vi "INI Create Semaphore.vi"(4 "error in":errorcluster) -> (0 "error out":errorcluster, 3 "semaphore":T1)   [LabVIEW 2013]
doc: "Produces the .ini semaphore that restricts reading/writing to the .ini file."
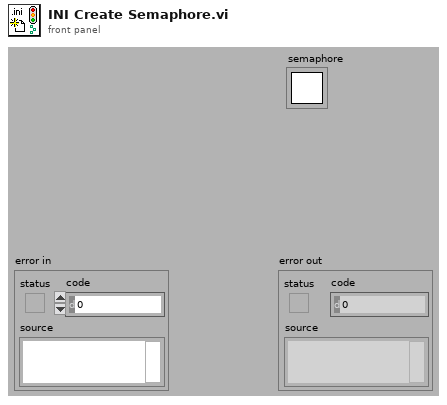
[diagram p1: front panel]
types:
  T1 = typedef "Semaphore RefNum" = refnum<k1>
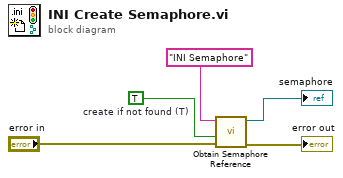
[diagram p0: block diagram]
diagram:
  w2 = TRUE  # create if not found (T)
  n1 = call <vilib>:"Obtain Semaphore Reference.vi"("error in (no error)"="error in", "create if not found (T)"=w2, "name (unnamed)"="INI Semaphore") -> ("error out"=→"error out":errorcluster, "semaphore"=→"semaphore":T1)  [unwired: 1 in, 2 out]
